vi "Get_SLOPE_data_from_file.vi"(11 "Output File Slopes Test":path=path "C:/KPRO_2010/Output_Files/Slopes.txt") -> (0 "Last_Pressure_Slope":dbl format="%.2f", 1 "Last_Flow_Slope":dbl format="%.2f", 2 "Last_String_Pot_Slope":dbl format="%.2f", 3 "Output_array":sgl[][](array[numeric]) format="%.2f")   [LabVIEW 2016]
uses:
  <vilib>/Utility/file.llb/Read From Spreadsheet File (DBL).vi
panel:
  out "Last_KPRO_Box_Number":dbl
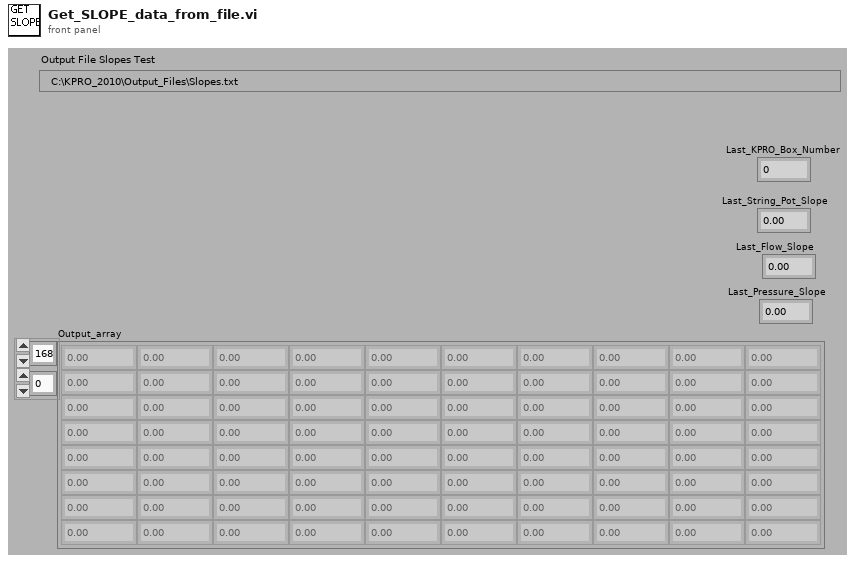
[diagram p1: front panel]
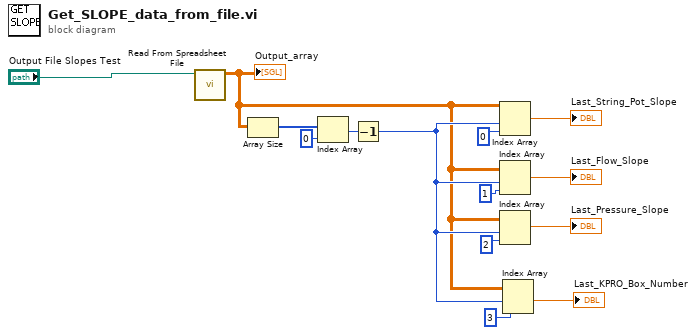
[diagram p0: block diagram]
diagram:
  n1 = call-poly <vilib>:"Read From Spreadsheet File.vi"("file path (dialog if empty)"="Output File Slopes Test") -> ("all rows"=w1:dbl[][])  [unwired: 6 in, 4 out]
  "Output_array" <- w1
  n2 = Array Size(array=w1) -> (size(s)=w13:i32[])
  n3 = Index Array(array=w13, index=0) -> (element=w12:i32)
  n4 = Decrement(x=w12) -> (x-1=w4:i32)
  n5 = Index Array(array=w1, index (row)=w4, index (col)=0 ("index")) -> (element=→"Last_String_Pot_Slope":dbl)
  n6 = Index Array(array=w1, index (row)=w4, index (col)=1 ("disabled index (col)")) -> (element=→"Last_Flow_Slope":dbl)
  n7 = Index Array(array=w1, index (row)=w4, index (col)=2 ("index")) -> (element=→"Last_Pressure_Slope":dbl)
  n8 = Index Array(array=w1, index (row)=w4, index (col)=3 ("index")) -> (element=→"Last_KPRO_Box_Number":dbl)
